vi "Move Chn to Wfm Canvas.vi"(7 "Channels Ctrl Ref":refnum<vi>, 8 "error in (no error)":errorcluster, 10 "Canvas Ctrl Refs":T1, 11 "To Save Wfm Arrays":waveform(dbl)[](array[waveform])) -> (0 "error out":errorcluster, 2 "Canvas Wfm Arrays":waveform(dbl)[](array[waveform]), 3 "Wfm Grp Data":T2)   [LabVIEW 2025, in "TDMS Waveform Creator UI.lvlib"]
uses:
  TDMS Waveform Creator UI.lvlib
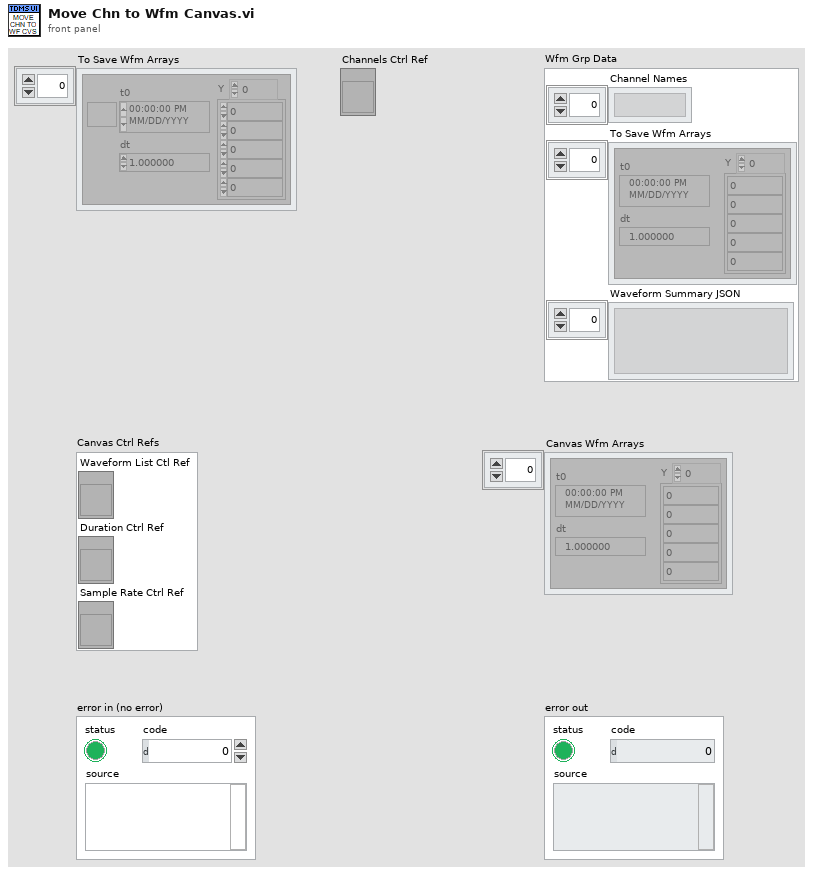
[diagram p1: front panel]
types:
  T1 = cluster{"Waveform List Ctl Ref":refnum<vi>, "Duration Ctrl Ref":refnum<vi>, "Sample Rate Ctrl Ref":refnum<vi>}
  T2 = cluster{"Channel Names":string[], "To Save Wfm Arrays":waveform(dbl)[], "Waveform Summary JSON":string[]}
  T3 = cluster{"Trim and Resample Settings":cluster{"Duration":dbl, "Sample Rate":dbl}, "Wfms Json":string[]}
  T4 = cluster{"Item Names":string[], waveform(dbl)[], string[]}
  T5 = cluster{"File Path":string, "Sample Rate (Hz)":dbl, "Read From":i32, "Pre Delay (s)":dbl, "Post Delay (s)":dbl, "Scale":dbl}
  T6 = cluster{"Waveform Type":i32, "Sample Rate (Hz)":dbl, "Frequency (Hz)":dbl, "Amplitude":dbl, "Number of Cycles":u32, "Ramp Start":dbl, "Ramp Stop":dbl, "Length (s)":dbl, "DC Value":dbl, "Duration (s)":dbl, "Pre Delay (s)":dbl, "Post Delay (s)":dbl}
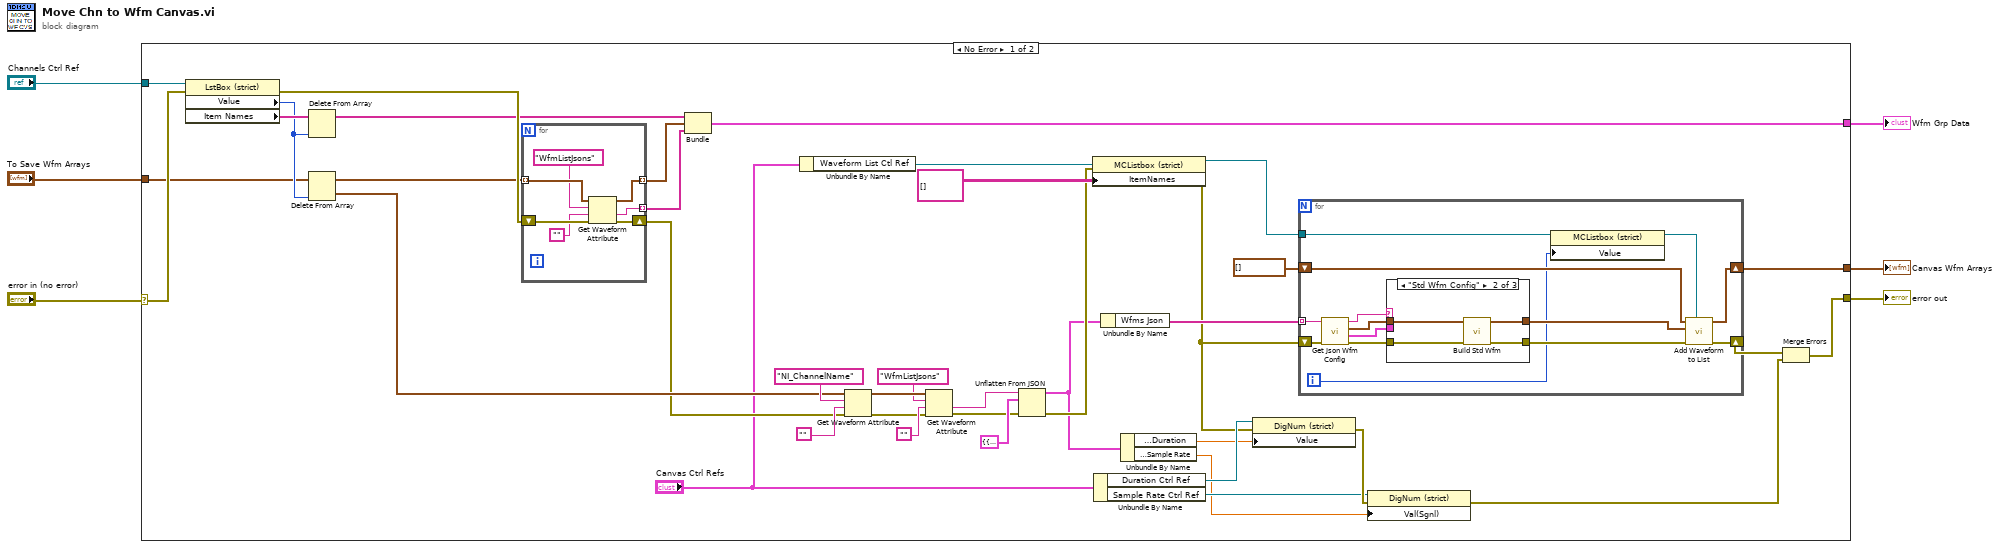
[diagram p0: block diagram]
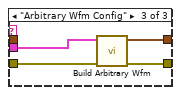
[diagram p3: hidden frame]
diagram:
  n1 = case shown="No Error" "error in (no error)" {
    selector: "error in (no error)" -> [w45 w77]
    tunnel: "Channels Ctrl Ref" -> [w46 _]
    tunnel: "To Save Wfm Arrays" -> [w41 _]
    tunnel: [w7 w77] -> w3
    tunnel: [w36 _] -> w2
    tunnel: [w23 _] -> w1
    frame No Error {
      n2 = property class="LstBox (strict)"(reference=w46, error in=w45) -> (error out=w44:errorcluster, "Value"=w42:i32, "Item Names"=w43:string[])  [unwired: 1 out]
      n3 = Delete From Array(array=w43, index=w42) -> (array with subset deleted=w39:string[])  [unwired: 1 in, 1 out]
      n4 = Delete From Array(array=w41, index=w42) -> (deleted portion=w32:waveform(dbl), array with subset deleted=w40:waveform(dbl)[])  [unwired: 1 in]
      n5 = for {
        shift-right: [w75] -> w25
        shift-left: w44 -> [w76]
        tunnel: w40 -> [w74] mode=indexing
        tunnel: [w73] -> w38 mode=indexing
        tunnel: [w70] -> w37 mode=indexing
        n6 = Get Waveform Attribute(4:w76, 5:"", 6:"WfmListJsons" ("name"), 7:w74) -> (0:w75:errorcluster, 1:w70:string, 3:w73:waveform(dbl))  [unwired: 1 out]
      }
      n7 = Bundle("Item Names"=w39, w38, w37) -> (w36:T4)  [unwired: 1 in]
      n8 = Unbundle By Name("Canvas Ctrl Refs") -> ("Waveform List Ctl Ref"=w21:refnum<vi>)
      n9 = Get Waveform Attribute(4:w25, 5:"", 6:"NI_ChannelName" ("name"), 7:w32) -> (0:w27:errorcluster, 3:w34:waveform(dbl))  [unwired: 2 out]
      n10 = Get Waveform Attribute(4:w27, 5:"", 6:"WfmListJsons" ("name"), 7:w34) -> (0:w28:errorcluster, 1:w30:string)  [unwired: 2 out]
      n11 = Unflatten From JSON(JSON string=w30, type and defaults=T3 {"Trim and Resample Settings"={"Duration"=0.0, "Sample Rate"=0.0}, "Wfms Json"=[]} ("Wfm Summary"), error in (no error)=w28) -> (value=w15:T3, error out=w18:errorcluster)  [unwired: 4 in]
      n12 = property class="MCListbox (strict)"(reference=w21, error in=w18, "ItemNames"=string[][] [] ("Item Names")) -> (reference out=w17:refnum<vi>, error out=w10:errorcluster)
      n13 = Unbundle By Name("Canvas Ctrl Refs") -> ("Duration Ctrl Ref"=w16:refnum<vi>, "Sample Rate Ctrl Ref"=w13:refnum<vi>)
      n14 = Unbundle By Name(w15) -> ("Wfms Json"=w24:string[])
      n15 = Unbundle By Name(w15) -> ("Trim and Resample Settings.Duration"=w12:dbl, "Trim and Resample Settings.Sample Rate"=w11:dbl)
      n16 = property class="DigNum (strict)"(reference=w16, error in=w10, "Value"=w12) -> (error out=w14:errorcluster)  [unwired: 1 out]
      n17 = for {
        tunnel: w24 -> [w60] mode=indexing
        shift-right: [w54] -> w9
        shift-left: w10 -> [w49]
        shift-right: [w52] -> w23
        shift-left: waveform(dbl)[] [] ("Waveform") -> [w53]
        tunnel: w17 -> [w50]
        i -> [w47]
        n18 = call "Get Json Wfm Config.vi"("error in"=w49, "Json String"=w60) -> ("error out"=w57:errorcluster, "Arbitrary Wfm Config"=w56:T5, "Std Wfm Config"=w58:T6, "Type"=w59:string)  [unwired: 6 in]
        n19 = case shown="\"Std Wfm Config\"" w59 {
          tunnel: w58 -> [_ w62 _]
          tunnel: w57 -> [w61 w65 w69]
          tunnel: w56 -> [_ _ w68]
          tunnel: [_ w63 w67] -> w51
          tunnel: [w61 w64 w66] -> w55
          frame Default {
          }
          frame "Std Wfm Config" {
            n20 = call "Build Std Wfm.vi"("error in"=w65, "Standard Wfm Config"=w62) -> ("error out"=w64:errorcluster, "Waveform"=w63:waveform(dbl))  [unwired: 6 in, 2 out]
          }
          frame "Arbitrary Wfm Config" {
            n21 = call "Build Arbitrary Wfm.vi"("error in"=w69, "Arbitrary Wfm Config"=w68) -> ("error out"=w66:errorcluster, "Waveform"=w67:waveform(dbl))  [unwired: 6 in, 2 out]
          }
        }
        n22 = property class="MCListbox (strict)"(reference=w50, "Value"=w47) -> (reference out=w48:refnum<vi>)  [unwired: 1 in, 1 out]
        n23 = call "Add Waveform to List.vi"("Waveform List Ctl Ref"=w48, "error in (no error)"=w55, "Waveform to Add"=w51, "Canvas Wfm Array In"=w53) -> ("error out"=w54:errorcluster, "Canvas Wfm Array Out"=w52:waveform(dbl)[])  [unwired: 6 in]
      }
      n24 = property class="DigNum (strict)"(reference=w13, error in=w14, "Val(Sgnl)"=w11) -> (error out=w8:errorcluster)  [unwired: 1 out]
      n25 = Merge Errors(w9, w8) -> (w7:errorcluster)
    }
    frame Error {
    }
  }
  "error out" <- w3
  "Wfm Grp Data" <- w2
  "Canvas Wfm Arrays" <- w1
